vi "Write WorkSpace.vi"(3 "(FPPos)":refnum<class "Frame_FPPos.lvclass">, 4 "WkSpace":T1) -> (5 "(FPPos) Out":refnum<class "Frame_FPPos.lvclass">)   [LabVIEW 2024, in "Frame_FPPos.lvclass"]
uses:
  Frame_FPPos.lvclass
  <vilib>/Utility/miscctls.llb/LVRectTypeDef.ctl
  Frame_FPPos.lvclass/Frame_FPPos.ctl
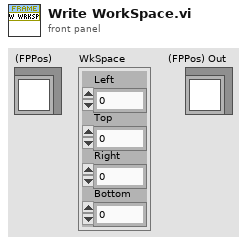
[diagram p1: front panel]
types:
  T1 = typedef "LVRectTypeDef.ctl" = cluster{"Left":i16, "Top":i16, "Right":i16, "Bottom":i16}
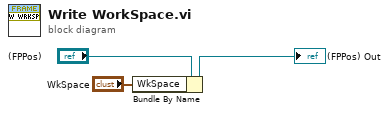
[diagram p0: block diagram]
diagram:
  n1 = Bundle By Name(cluster="(FPPos)", "WkSpace"="WkSpace") -> (→"(FPPos) Out":refnum<class "Frame_FPPos.lvclass">)
